vi "SrvStart.vi"(0 "ref in":u64, 11 "error in (no error)":errorcluster) -> (4 "ref out":u64, 6 "return type":i32, 15 "error out":errorcluster)   [LabVIEW 2010, in "Snap7.lvlib"]
uses:
  Snap7.lvlib
  windows/lv_snap7.dll
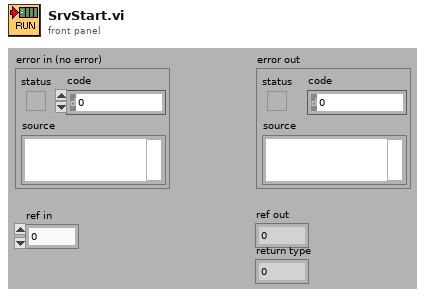
[diagram p1: front panel]
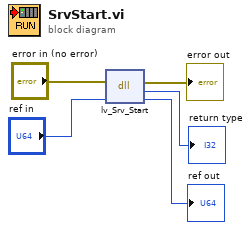
[diagram p0: block diagram]
diagram:
  n1 = dll-call lib="C:/snap7-src-1.0.0/LabVIEW/lib/windows/lv_snap7.dll" fn="lv_Srv_Start"(error in="error in (no error)", "Server"="ref in") -> (error out=→"error out":errorcluster, "return type"=→"return type":i32, "Server"=→"ref out":u64)  [unwired: 2 in, 1 out]
